vi "CRYWindow Close.vi"   [LabVIEW 2013]
panel:
  # "Close window"
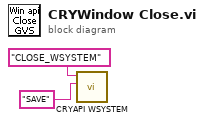
[diagram p0: block diagram]
diagram:
  n1 = call "CRYAPI WSYSTEM.vi"("sOption"="SAVE" ("sData"), "sAction"="CLOSE_WSYSTEM") -> ()  [unwired: 2 in, 8 out]
